vi "DAC8568_sendData.vi"(6 "feature":u8, 7 "data":u16, 8 "error in (no error)":errorcluster, 9 "addr":u8, 10 "ctrl":u8, 11 "location":u8) -> (0 "error out":errorcluster)   [LabVIEW 2015, in "ESLSCDLL.lvlib"]
uses:
  ESLSCDLL.lvlib
  Globals.vi
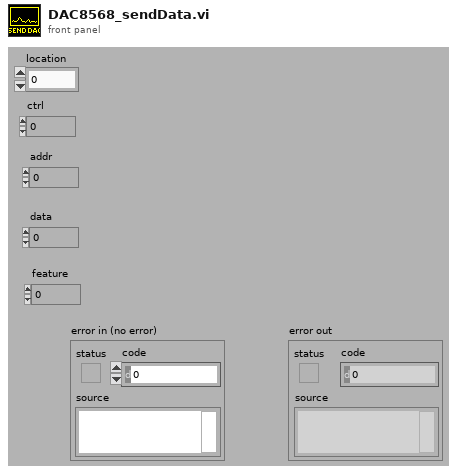
[diagram p1: front panel]
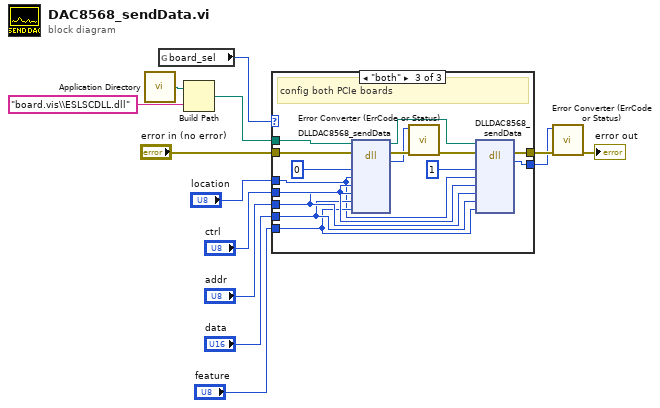
[diagram p0: block diagram]
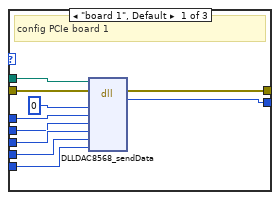
[diagram p2: hidden frame]
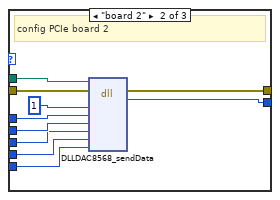
[diagram p3: hidden frame]
diagram:
  n1 = call <vilib>:"Application Directory.vi"() -> ("Application Directory"=w4:path)
  n2 = global read "Globals.vi" "board_sel"() -> (w5:enum16{"0", "board 1", "board 2", "both"})
  n3 = Build Path(base path=w4, name or relative path="board.vis\\ESLSCDLL.dll") -> (appended path=w2:path)
  n4 = case shown="\"both\"" w5 {
    tunnel: "feature" -> [w23 w30 w43]
    tunnel: "data" -> [w22 w31 w44]
    tunnel: "addr" -> [w21 w32 w45]
    tunnel: "ctrl" -> [w20 w33 w46]
    tunnel: "error in (no error)" -> [w19 w29 w37]
    tunnel: [w18 w28 w39] -> w7
    tunnel: [w17 w27 w38] -> w6
    tunnel: w2 -> [w16 w26 w36]
    tunnel: "location" -> [w15 w25 w34]
    frame "board 1", Default {
      # "config PCIe board 1"
      n5 = dll-call lib="C:/ENTW/PCIE/LV64/board.vis/ESLSCDLL.dll" fn="DLLDAC8568_sendData" ("lwlscdll.dll:DLLSetADAmpRed")(path in=w16, error in=w19, "drvno"=u32 0, "location"=w15, "ctrl"=w20, "addr"=w21, "data"=w22, "feature"=w23) -> (error out=w18:errorcluster, "es_status_codes"=w17:i32)  [unwired: 7 in, 1 out]
    }
    frame "board 2" {
      # "config PCIe board 2"
      n6 = dll-call lib="C:/ENTW/PCIE/LV64/board.vis/ESLSCDLL.dll" fn="DLLDAC8568_sendData" ("lwlscdll.dll:DLLSetADAmpRed")(path in=w26, error in=w29, "drvno"=u32 1, "location"=w25, "ctrl"=w33, "addr"=w32, "data"=w31, "feature"=w30) -> (error out=w28:errorcluster, "es_status_codes"=w27:i32)  [unwired: 7 in, 1 out]
    }
    frame "both" {
      # "config both PCIe boards"
      n7 = dll-call lib="C:/ENTW/PCIE/LV64/board.vis/ESLSCDLL.dll" fn="DLLDAC8568_sendData" ("lwlscdll.dll:DLLSetADAmpRed")(path in=w36, error in=w37, "drvno"=u32 0, "location"=w34, "ctrl"=w46, "addr"=w45, "data"=w44, "feature"=w43) -> (path out=w35:path, error out=w42:errorcluster, "es_status_codes"=w41:i32)  [unwired: 7 in]
      n8 = call "Error Converter (ErrCode or Status).vi"("error in (no error)"=w42, "error code"=w41) -> ("error out"=w40:errorcluster)  [unwired: 9 in]
      n9 = dll-call lib="C:/ENTW/PCIE/LV64/board.vis/ESLSCDLL.dll" fn="DLLDAC8568_sendData" ("lwlscdll.dll:DLLSetADAmpRed")(path in=w35, error in=w40, "drvno"=u32 1, "location"=w34, "ctrl"=w46, "addr"=w45, "data"=w44, "feature"=w43) -> (error out=w39:errorcluster, "es_status_codes"=w38:i32)  [unwired: 7 in, 1 out]
    }
  }
  n10 = call "Error Converter (ErrCode or Status).vi"("error in (no error)"=w7, "error code"=w6) -> ("error out"=→"error out":errorcluster)  [unwired: 9 in]
